vi "passTestThreadOrganizer.vi"(6 "Pass intercepted":T1, 7 "Maintains ball possesion?":T1, 8 "Ball missed robot":T1, 9 "Robot kicks ball":T1, 10 "Ball out":T1, 11 "Ball stops":T1) -> (1 "Pass state":T2, 2 "Result":T1, 3 "Result":T1)   [LabVIEW 2017]
uses:
  passTestStates.ctl
  <extravilib>/ChannelInstances/Lossy Stream-t'passTestStates.ctl'/)Channel.ctl
  <extravilib>/ChannelInstances/Lossy Stream-t'passTestStates.ctl'/Write With Abort.vi
  <extravilib>/ChannelInstances/Lossy Stream-t'passTestStates.ctl'/Read With Abort.vi
  <extravilib>/ChannelInstances/Lossy Stream-t'passTestStates.ctl'/Endpoint.vi
  <extravilib>/ChannelInstances/Lossy Stream-t'passTestStates.ctl'/EndpointRead.vi
  <extravilib>/ChannelInstances/Lossy Stream-t'passTestStates.ctl'/)Channel.vi
  <resource>/ChannelSupport/_ChannelSupport/WaitIfNeeded.vi
  SOS/passTestAllResults.vi
  SOS/passStateGlobalVariableResult.vi
  <extravilib>/ChannelInstances/Lossy Stream-t'passTestStates.ctl'.lvlib
panel:
  out "Array":T2[](array[typedef])
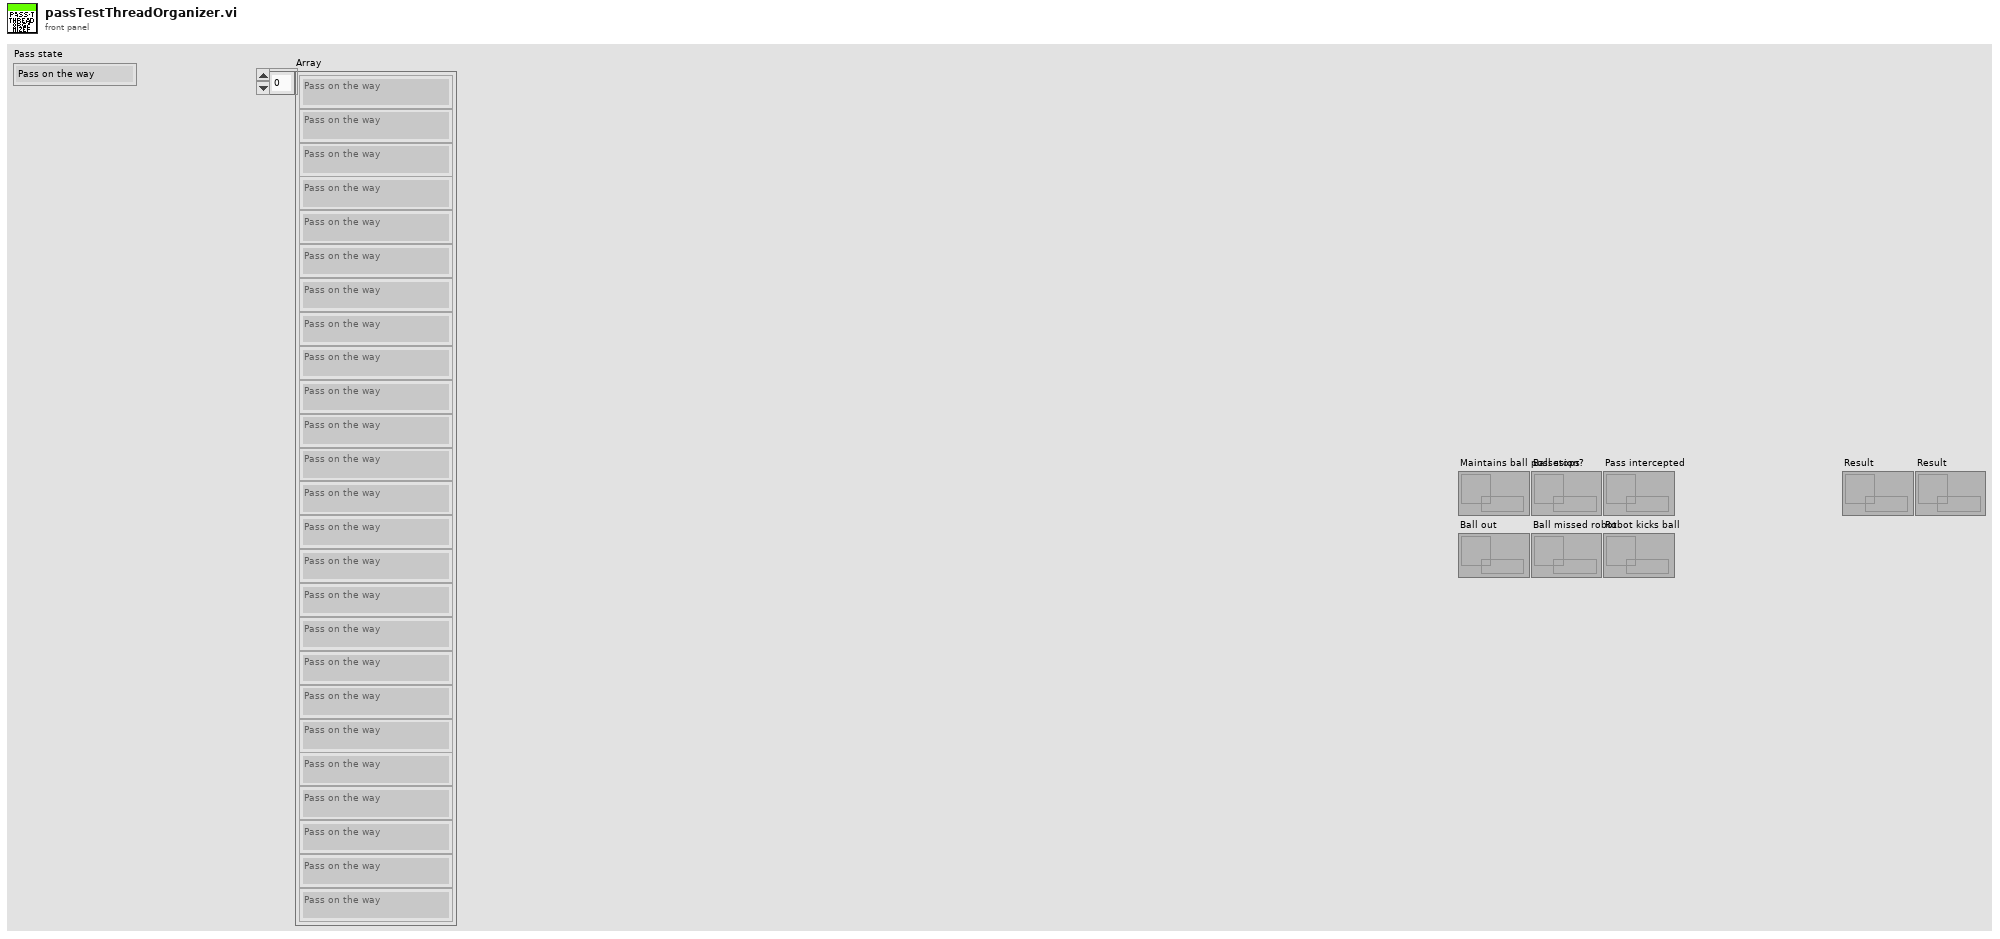
[diagram p1: front panel]
types:
  T1 = typedef "Lossy Stream-t'passTestStates.ctl'.lvlib/)Channel.ctl" = refnum<queue>
  T2 = typedef "passTestStates.ctl" = enum16{"Pass on the way", "Ball stops", "Pass intercepted", "Ball out of the field", "Ball missed robot", "Need more force to pass", "Too much force", "Correct pass", "Keep ball possesion", "Robot kicked the ball", "Waiting Kick", "Invalid: same robot", "Invalid: kicker ID 999", "Invalid: Receiver ID 999", "Invalid"}
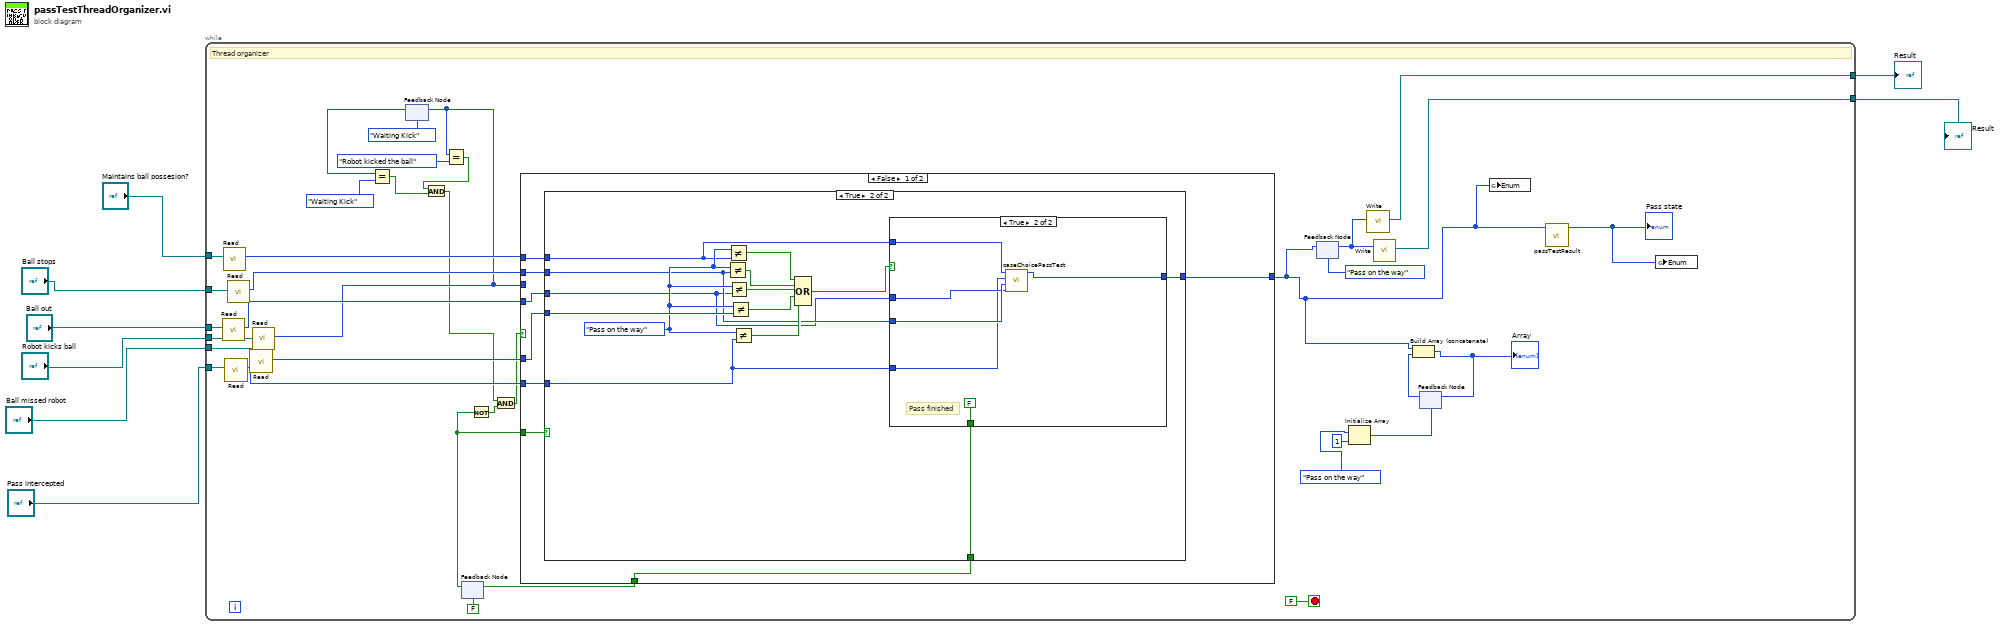
[diagram p0: block diagram]
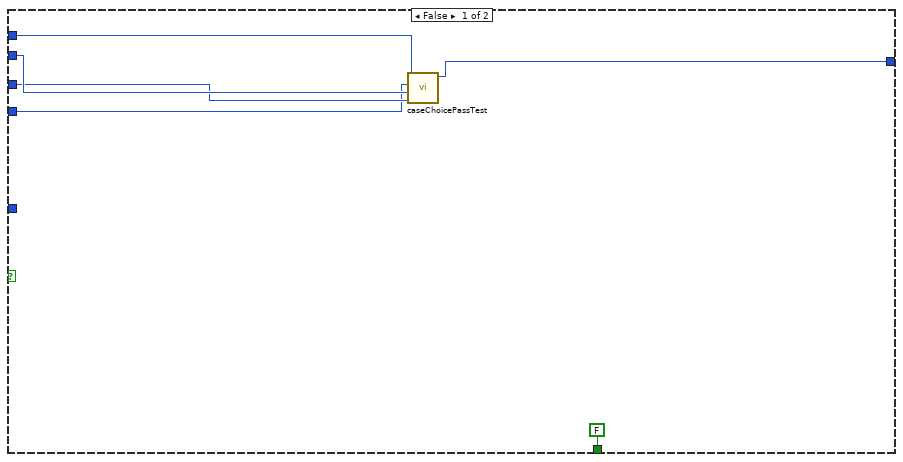
[diagram p2: hidden frame]
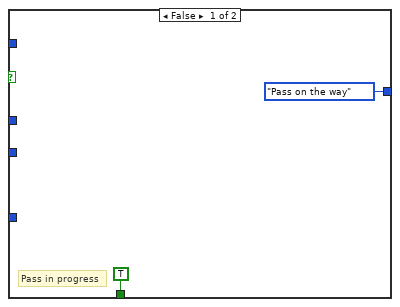
[diagram p3: hidden frame]
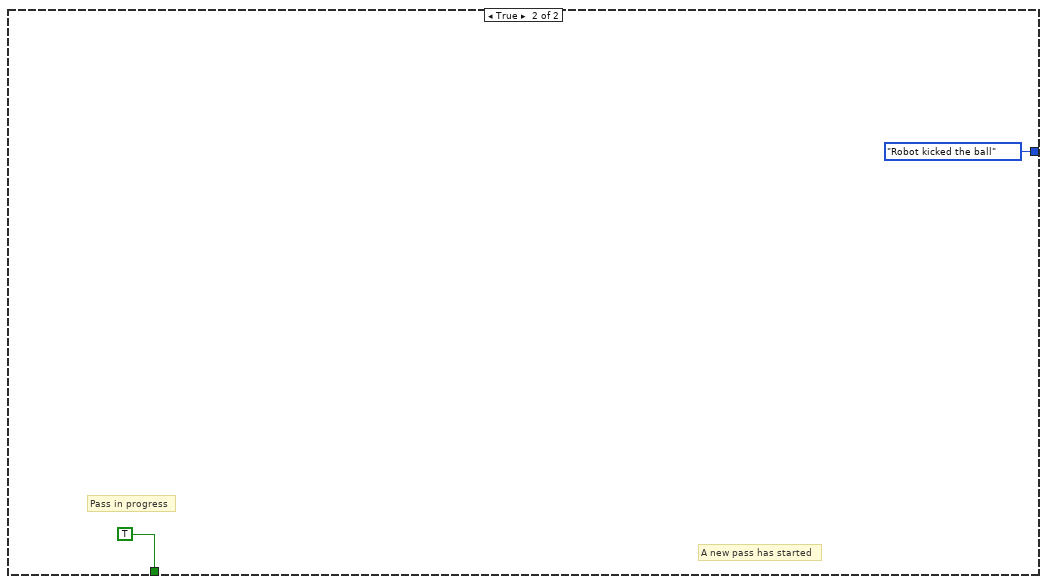
[diagram p4: hidden frame]
diagram:
  n1 = while {
    tunnel: "Pass intercepted" -> [w38]
    tunnel: "Ball missed robot" -> [w39]
    tunnel: "Ball out" -> [w41]
    tunnel: "Ball stops" -> [w42]
    tunnel: "Maintains ball possesion?" -> [w43]
    tunnel: "Robot kicks ball" -> [w40]
    tunnel: [w12] -> w2
    tunnel: [w11] -> w1
    stop <- FALSE stop-if-true
    # "Thread organizer"
    n2 = call <extravilib>:"Read.vi"("channel"=w41) -> ("element"=w34:T2)  [unwired: 5 in, 5 out]
    n3 = call <extravilib>:"Read.vi"("channel"=w43) -> ("element"=w36:T2)  [unwired: 5 in, 5 out]
    n4 = call <extravilib>:"Read.vi"("channel"=w38) -> ("element"=w32:T2)  [unwired: 5 in, 5 out]
    n5 = call <extravilib>:"Read.vi"("channel"=w42) -> ("element"=w35:T2)  [unwired: 5 in, 5 out]
    n6 = call <extravilib>:"Read.vi"("channel"=w39) -> ("element"=w33:T2)  [unwired: 5 in, 5 out]
    n7 = call <extravilib>:"Read.vi"("channel"=w40) -> ("element"=w26:T2)  [unwired: 5 in, 5 out]
    n8 = feedback-in #1(w26) -> ()
    n9 = feedback #1(passTestStates."Waiting Kick" ("element")) -> (w31:T2)
    n10 = Equal?(x=w31, y=passTestStates."Waiting Kick") -> (x = y?=w29:bool)
    n11 = Equal?(x=w26, y=passTestStates."Robot kicked the ball") -> (x = y?=w27:bool)
    n12 = And(x=w27, y=w29) -> (x .and. y?=w22:bool)
    n13 = feedback #2(FALSE) -> (w21:bool)
    n14 = Not(x=w21) -> (.not. x?=w24:bool)
    n15 = And(x=w22, y=w24) -> (x .and. y?=w20:bool)
    n16 = case shown="False" w20 {
      tunnel: w26 -> [_ _]
      tunnel: w36 -> [w52 _]
      tunnel: w35 -> [w51 _]
      tunnel: w34 -> [w50 _]
      tunnel: w33 -> [w49 _]
      tunnel: w32 -> [w48 _]
      tunnel: [w47 TRUE] -> w23
      tunnel: w21 -> [w46 _]
      tunnel: [w45 passTestStates."Robot kicked the ball" ("Result")] -> w9
      frame False {
        n17 = case shown="True" w46 {
          tunnel: w52 -> [w57 w63]
          tunnel: w51 -> [w56 w62]
          tunnel: w50 -> [w55 w61]
          tunnel: w49 -> [w54 w72]
          tunnel: w48 -> [_ w60]
          tunnel: [FALSE w64] -> w47
          tunnel: [w53 w59] -> w45
          frame False {
            n18 = call "caseChoicePassTest.vi"("Out of the field"=w55, "Ball stops"=w56, "Pass intercepted"=w54, "Too much force\nCorrect pass\nKeep ball possesion\nInvalid Situation\nPass on the way"=w57) -> ("Result"=w53:T2)  [unwired: 7 in]
          }
          frame True {
            w71 = passTestStates."Pass on the way" ("element")
            n19 = Not Equal?(x=w71, y=w62) -> (x != y?=w69:bool)
            n20 = Not Equal?(x=w71, y=w63) -> (x != y?=w70:bool)
            n21 = Not Equal?(x=w71, y=w61) -> (x != y?=w68:bool)
            n22 = Not Equal?(x=w71, y=w72) -> (x != y?=w67:bool)
            n23 = Not Equal?(x=w71, y=w60) -> (x != y?=w66:bool)
            n24 = Compound Arithmetic op=OR(w70, w69, w68, w67, w66) -> (w65:bool)
            n25 = case shown="True" w65 {
              tunnel: [TRUE FALSE] -> w64
              tunnel: w63 -> [_ w79]
              tunnel: w62 -> [_ w78]
              tunnel: w61 -> [_ w77]
              tunnel: w60 -> [_ w76]
              tunnel: [passTestStates."Pass on the way" ("Result") w75] -> w59
              frame False {
                # "Pass in progress"
              }
              frame True {
                # "Pass finished"
                n26 = call "caseChoicePassTest.vi"("Out of the field"=w77, "Ball stops"=w78, "Pass intercepted"=w76, "Too much force\nCorrect pass\nKeep ball possesion\nInvalid Situation\nPass on the way"=w79) -> ("Result"=w75:T2)  [unwired: 7 in]
              }
            }
          }
        }
      }
      frame True {
        # "Pass in progress"
        # "A new pass has started"
      }
    }
    n27 = feedback-in #2(w23) -> ()
    n28 = feedback #3(passTestStates."Pass on the way" ("Result")) -> (w18:T2)
    n29 = feedback-in #3(w9) -> ()
    n30 = Initialize Array(passTestStates."Pass on the way" ("Result"), 1 ("dimension size")) -> (w13:T2[])
    n31 = call <extravilib>:"Write.vi"("element"=w18) -> ("channel"=w12:T1)  [unwired: 8 in, 2 out]
    n32 = call <extravilib>:"Write.vi"("element"=w18) -> ("channel"=w11:T1)  [unwired: 8 in, 2 out]
    n33 = feedback #4(w13) -> (w14:T2[])
    n34 = Build Array (concatenate)(w9, w14) -> (w15:T2[])
    "Array" <- w15
    n35 = feedback-in #4(w15) -> ()
    n36 = global write "passTestAllResults.vi" "Enum"(w9) -> ()
    n37 = call "passTestResult.vi"("State"=w9) -> ("Pass state"=w10:T2)  [unwired: 10 in]
    "Pass state" <- w10
    n38 = global write "passStateGlobalVariableResult.vi" "Enum"(w10) -> ()
  }
  "Result" <- w2
  "Result" <- w1
